vi "Device_selection.vi"(10 "error in (no error)":errorcluster, 11 "device count":u8) -> (2 "error out":errorcluster, 3 "Loop Tunnel":i32)   [LabVIEW 2026]
panel:
  out "Number of Devices":string[](array[string])
  out "Status":string[](array[string])
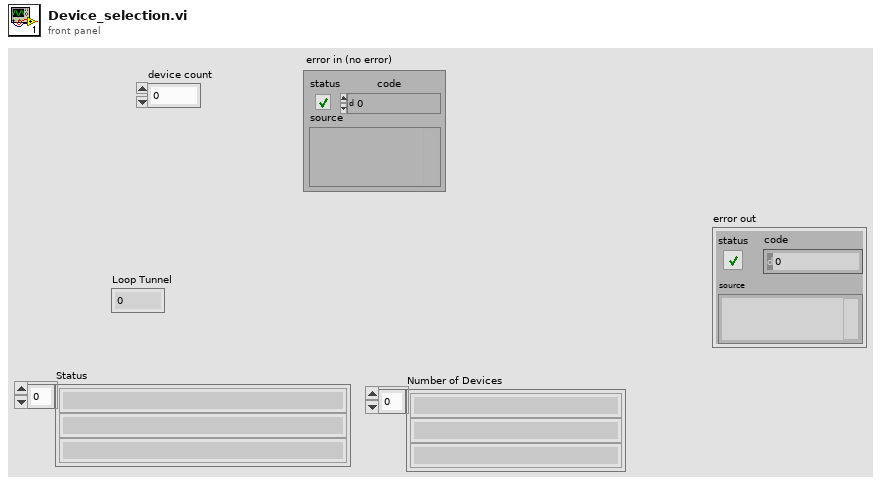
[diagram p1: front panel]
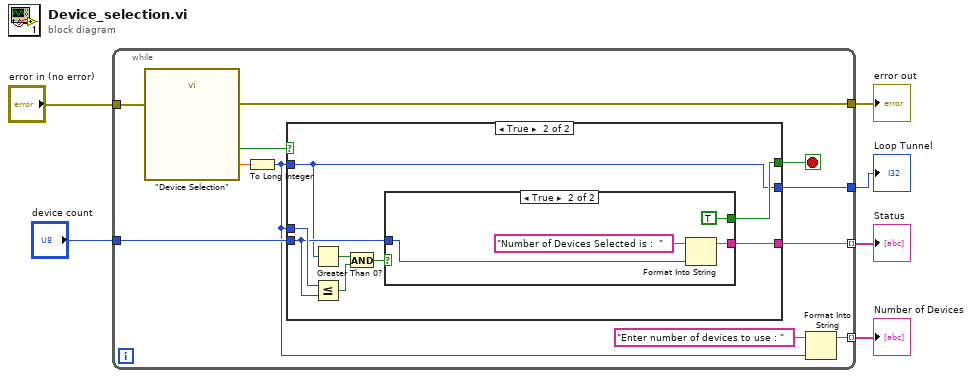
[diagram p0: block diagram]
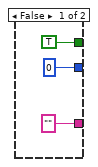
[diagram p2: hidden frame]
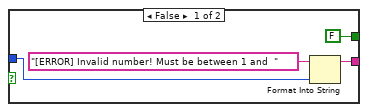
[diagram p3: hidden frame]
diagram:
  n1 = while {
    tunnel: "device count" -> [w16]
    tunnel: [w15] -> w6 mode=indexing
    tunnel: [w12] -> w4
    tunnel: [w10] -> w5 mode=indexing
    tunnel: [w9] -> w3
    tunnel: "error in (no error)" -> [w7]
    stop <- w14 stop-if-true
    n2 = call "\"Device Selection\""("error in (no error)"=w7) -> ("\"Device Count\""=w11:dbl, "OK"=w17:bool, "error out"=w9:errorcluster)  [unwired: 16 in]
    n3 = To Long Integer(number=w11) -> (32bit integer=w8:i32)
    n4 = case shown="True" w17 {
      tunnel: w8 -> [_ w21]
      tunnel: w8 -> [_ w26]
      tunnel: w16 -> [_ w24]
      tunnel: [TRUE w23] -> w14
      tunnel: ["" w22] -> w15
      tunnel: [0 w21] -> w12
      frame False {
      }
      frame True {
        n5 = Greater Than 0?(x=w21) -> (x > 0?=w27:bool)
        n6 = Less Or Equal?(x=w26, y=w24) -> (x <= y?=w28:bool)
        n7 = And(x=w27, y=w28) -> (x .and. y?=w25:bool)
        n8 = case shown="True" w25 {
          tunnel: w24 -> [w32 w35]
          tunnel: [FALSE TRUE] -> w23
          tunnel: [w29 w33] -> w22
          frame False {
            n9 = Format Into String(initial string="[ERROR] Invalid number! Must be between 1 and  ", w32) -> (resulting string=w29:string)  [unwired: 2 in, 1 out]
          }
          frame True {
            n10 = Format Into String(initial string="Number of Devices Selected is :  ", w35) -> (resulting string=w33:string)  [unwired: 2 in, 1 out]
          }
        }
      }
    }
    n11 = Format Into String(initial string="Enter number of devices to use : ", w8) -> (resulting string=w10:string)  [unwired: 2 in, 1 out]
  }
  "Status" <- w6
  "Number of Devices" <- w5
  "Loop Tunnel" <- w4
  "error out" <- w3
